vi "Get Plot at Mouse Click [AC].vi"(8 "error in (no error)":errorcluster, 10 "Mouse Click Coordinates":T1, 11 "XY Graph":refnum<vi>) -> (0 "error out":errorcluster, 1 "Click is in Legend?":bool, 2 "Plot at Coordinates":i32, 3 "XY Graph":refnum<vi>)   [LabVIEW 2021, in "Graphs.lvlib"]
uses:
  Graphs.lvlib
  <vilib>/Utility/miscctls.llb/LVPoint32TypeDef.ctl
  Get Plot at Mouse Click in Plot Area [AC].vi
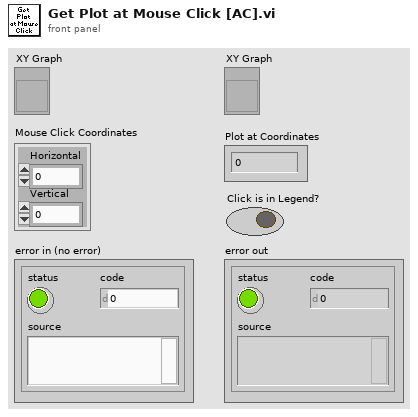
[diagram p1: front panel]
types:
  T1 = typedef "LVPoint32TypeDef.ctl" = cluster{"Horizontal":i32, "Vertical":i32}
  T2 = typedef "LVPositionTypeDef.ctl" = cluster{"Left":i32, "Top":i32}
  T3 = typedef "LVBoundsTypeDef.ctl" = cluster{"Width":u32, "Height":u32}
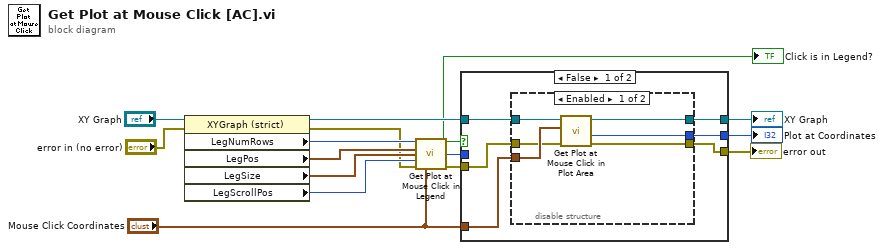
[diagram p0: block diagram]
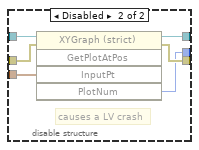
[diagram p2: hidden frame]
diagram:
  n1 = property class="XYGraph (strict)"(reference="XY Graph", error in="error in (no error)") -> (reference out=w10:refnum<vi>, error out=w2:errorcluster, "LegNumRows"=w11:u32, "LegPos"=w7:T2, "LegSize"=w6:T3, "LegScrollPos"=w5:u32)
  n2 = call "Get Plot at Mouse Click in Legend.vi"("LegNumRows"=w11, "Legend:Position"=w7, "Legend:Size"=w6, "LegScrollPos"=w5, "Error In"=w2, "Mouse Click Coordinates"="Mouse Click Coordinates") -> ("Click is in Legend?"=w9:bool, "Plot Index"=w3:i32, "Error Out"=w1:errorcluster)  [unwired: 7 in]
  "Click is in Legend?" <- w9
  n3 = case shown="False" w9 {
    tunnel: w10 -> [w18 w36]
    tunnel: [w21 w36] -> w12
    tunnel: w3 -> [_ w35]
    tunnel: [w20 w35] -> w13
    tunnel: "Mouse Click Coordinates" -> [w19 _]
    tunnel: w1 -> [w17 w34]
    tunnel: [w16 w34] -> w15
    frame False {
      n4 = disable-structure shown="Enabled" {
        disable-tunnel: [w27 w32] -> w21
        disable-tunnel: [w26 w28] -> w20
        disable-tunnel: w19 -> [w25 w30]
        disable-tunnel: w18 -> [w24 w33]
        disable-tunnel: w17 -> [w23 w31]
        disable-tunnel: [w22 w29] -> w16
        frame Enabled {
          n5 = call-poly "Get Plot at Mouse Click in Plot Area.vi"("error in (no error)"=w23, "Mouse Click Coordinates"=w25, "XY Graph"=w24) -> ("error out"=w22:errorcluster, "Plot Index"=w26:i32, "XY Graph"=w27:refnum<vi>)  [unwired: 6 in]
        }
        frame Disabled {
          # "causes a LV crash"
          n6 = invoke class="XYGraph (strict)" method="GetPlotAtPos"(reference=w33, error in=w31, "InputPt"=w30) -> (reference out=w32:refnum<vi>, error out=w29:errorcluster, "PlotNum"=w28:i32)  [unwired: 2 in, 2 out]
        }
      }
    }
    frame True {
      # "In the Legend Region"
    }
  }
  "error out" <- w15
  "Plot at Coordinates" <- w13
  "XY Graph" <- w12
